vi "set user settings.vi"(8 "error in (no error)":errorcluster, 9 "user settings":T1, 10 "id":string, 11 "DSFConfiguration in":refnum<class "DSFConfiguration.lvclass">) -> (0 "error out":errorcluster, 3 "DSFConfiguration out":refnum<class "DSFConfiguration.lvclass">)   [LabVIEW 2017, in "DSFConfiguration.lvclass"]
uses:
  DSFConfiguration.lvclass
  IDable/IDable.lvclass
  DSFPluginSettings/DSFPluginSettings.lvclass
  C:/github/data-sharing-framework-custom-device/Source/Submodules/DSF/Source/Configuration API/Classes/IDable/IDable.lvclass
  Controls/dsf configuration file/1.0.0/dsf settings.ctl
  Controls/dsf configuration file/1.0.0/dsf configuration file v1.0.0.lvlib
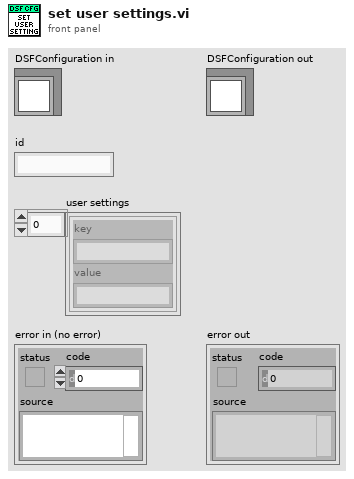
[diagram p1: front panel]
types:
  T1 = typedef "dsf configuration file v1.0.0.lvlib/dsf settings.ctl" = cluster{"key":string, "value":string}[]
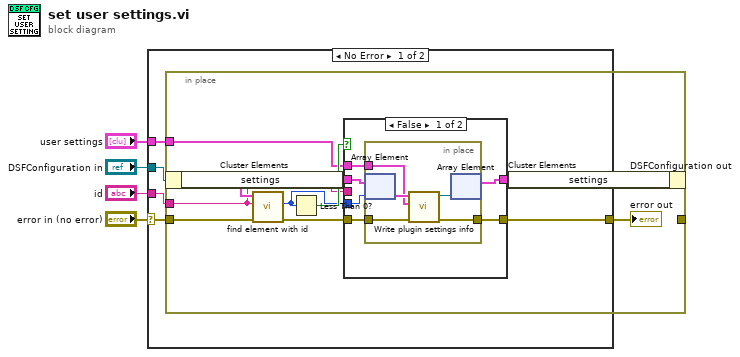
[diagram p0: block diagram]
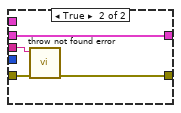
[diagram p2: hidden frame]
diagram:
  n1 = case shown="No Error" "error in (no error)" {
    selector: "error in (no error)" -> [w10 w38]
    tunnel: [w8 w38] -> w5
    tunnel: [w9 w37] -> w3
    tunnel: "DSFConfiguration in" -> [w12 w37]
    tunnel: "id" -> [w11 _]
    tunnel: "user settings" -> [w7 _]
    frame No Error {
      n2 = in-place {
        in-place-border: w11 -> [w13]
        in-place-border: w10 -> [w21]
        in-place-border: [w18] -> w8
        in-place-border: w7 -> [w15]
        n3 = in-place-cluster #1(w12) -> ("settings"=w17:cluster{"id":string, "values":T1}[])
        n4 = call "find element with id.vi"("error in (no error)"=w21, "id"=w13, "IDable Array in"=w17) -> ("error out"=w19:errorcluster, "index"=w16:i32)  [unwired: 7 in]
        n5 = Less Than 0?(x=w16) -> (x < 0?=w20:bool)
        n6 = case shown="False" w20 {
          tunnel: w19 -> [w24 w33]
          tunnel: [w23 w36] -> w18
          tunnel: w17 -> [w27 w35]
          tunnel: w16 -> [w26 _]
          tunnel: w15 -> [w25 _]
          tunnel: [w22 w35] -> w14
          tunnel: w13 -> [_ w34]
          frame False {
            n7 = in-place {
              in-place-border: w25 -> [w28]
              in-place-border: w24 -> [w32]
              in-place-border: [w31] -> w23
              n8 = in-place-array #2(w27, w26) -> (w30:cluster{"id":string, "values":T1})
              n9 = call "Write plugin settings info.vi"("error in (no error)"=w32, "plugin settings info"=w28, "DSFPluginSettings in"=w30) -> ("error out"=w31:errorcluster, "DSFPluginSettings out"=w29:refnum<class "DSFPluginSettings.lvclass">)  [unwired: 7 in]
              n10 = in-place-array #2(w29) -> (w22:cluster{"id":string, "values":T1}[])  [unwired: 1 out]
            }
          }
          frame True {
            n11 = call "throw not found error.vi"("error in (no error)"=w33, "id"=w34) -> ("error out"=w36:errorcluster)  [unwired: 9 in]
          }
        }
        n12 = in-place-cluster #1("settings"=w14) -> (w9:refnum<class "DSFConfiguration.lvclass">)
      }
    }
    frame Error {
    }
  }
  "error out" <- w5
  "DSFConfiguration out" <- w3
